vi "AI Regs Group UI.vi"(8 "error in (no error)":errorcluster, 11 "Node Ptr":T2 format="%.0x") -> (0 "error out":errorcluster)   [LabVIEW 2021, in "Modbus Master System Explorer.lvlib"]
uses:
  Modbus Master System Explorer.lvlib
  <vilib>/NI VeriStand/Custom Device API/Custom Device Item Ref.ctl
  SubVIs/Conflict Table.ctl
  SubVIs/Modbus Type.ctl
  <vilib>/NI VeriStand/Custom Device API/Custom Device API.lvlib
  <vilib>/NI VeriStand/Custom Device Tools/Custom Device Utility Library/Custom Device Utility Library.lvlib
  Shared/Modbus Master Shared.lvlib
panel:
  in  "Delete Multiple":bool
  in  "Add One":bool
  in  "Bulk Add":bool
  out "Conflicting Input Register Mappings":T1
  in  "Header":cluster{"Section Name":string}={"Section Name"="Input Register Group Settings"}
  in  "Description":string
  in  "Name":string
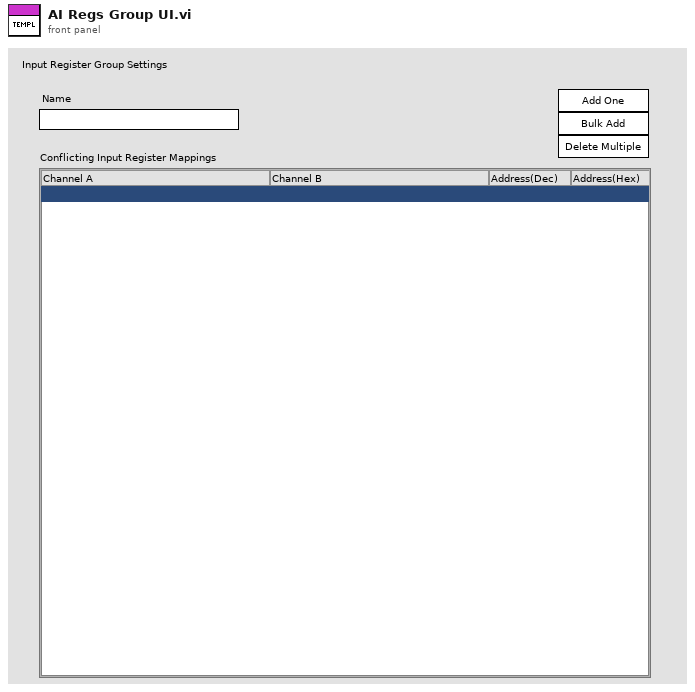
[diagram p1: front panel]
types:
  T1 = typedef "Modbus Master System Explorer.lvlib/Conflict Table.ctl" = i32
  T2 = typedef "Custom Device API.lvlib/Custom Device Item Ref.ctl" = u64
  T3 = typedef "Modbus Master Shared.lvlib/Modbus Type.ctl" = enum16{"Coil", "Discrete Input", "Holding Register", "Input Register"}
  T4 = typedef "Custom Device API.lvlib/Custom Device Item Info.ctl" = cluster{"Name":string, "Is Channel":bool, "GUID":string, "Is Waveform":bool}
  T5 = cluster{"Name":string, "Name":string, "Mapping":u16}[]
  T6 = typedef "Custom Device API.lvlib/Custom Device Commands.ctl" = enum16{"Default", "Item renamed", "Shutdown", "Dynamic button pressed"}
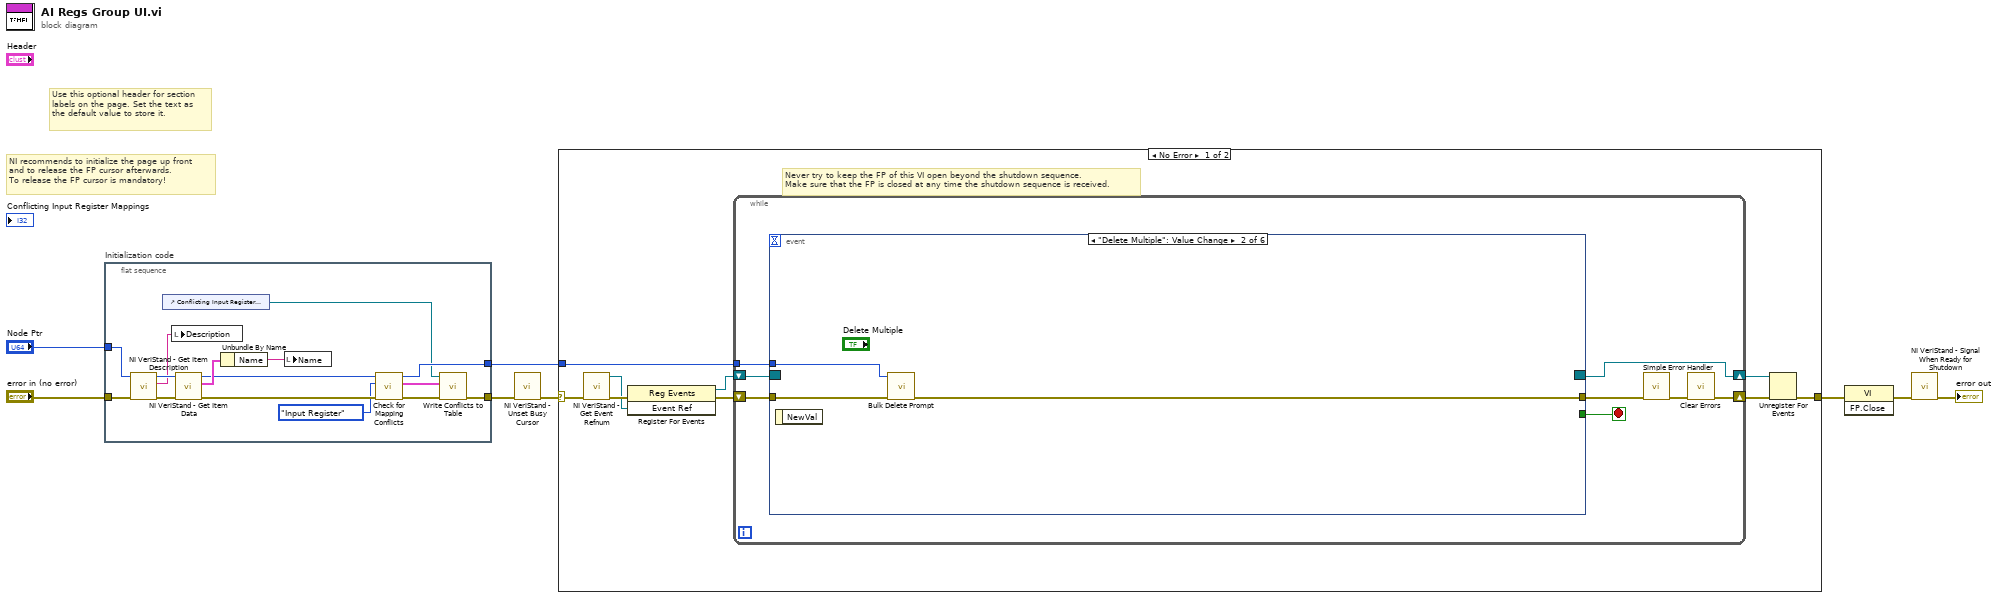
[diagram p0: block diagram]
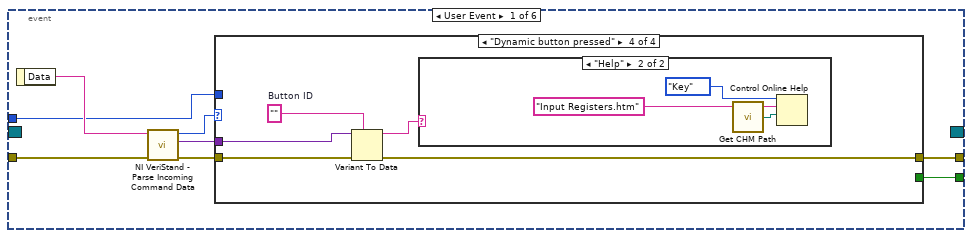
[diagram p2: hidden frame]
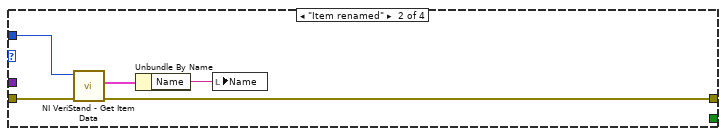
[diagram p4: hidden frame]
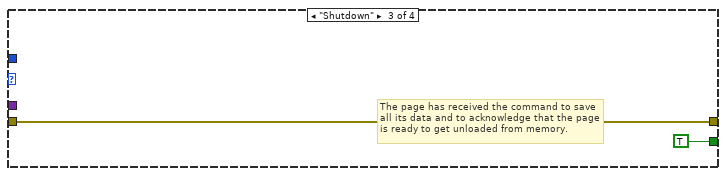
[diagram p5: hidden frame]
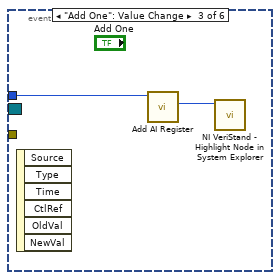
[diagram p7: hidden frame]
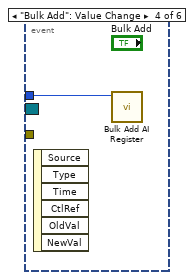
[diagram p8: hidden frame]
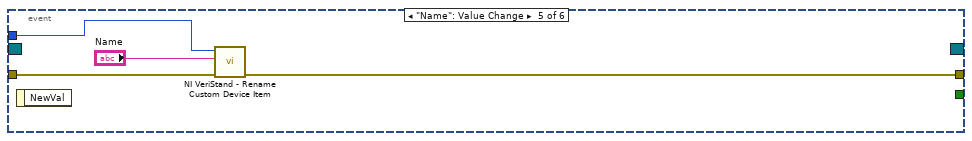
[diagram p9: hidden frame]
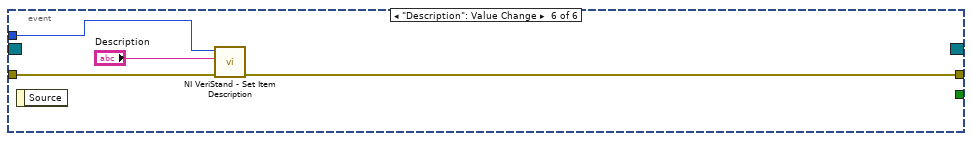
[diagram p10: hidden frame]
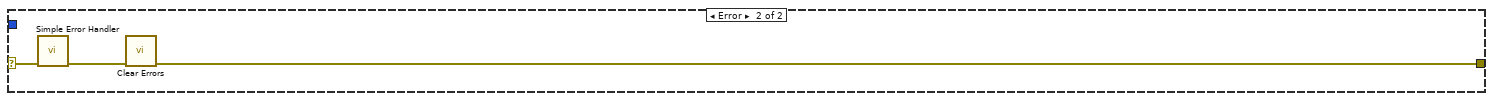
[diagram p11: hidden frame]
diagram:
  # "Use this optional header for section labels on the page. Set the text as the default value to store it."
  # "NI recommends to initialize the page up front\nand to release the FP cursor afterwards.\nTo release the FP cursor is mandatory!"
  n1 = flat-sequence "Initialization code" {
    tunnel: "error in (no error)" -> [w22]
    tunnel: "Node Ptr" -> [w21]
    tunnel: [w10] -> w4
    tunnel: [w15] -> w1
    frame #0 {
      n2 = call <vilib>:"NI VeriStand - Get Item Description.vi"("error in (no error)"=w22, "Item Ref in"=w21) -> ("error out"=w19:errorcluster, "Description"=w20:string, "Item Ref out"=w23:T2)  [unwired: 7 out]
      n3 = control-ref of="Conflicting Input Register Mappings"() -> (w13:refnum<vi>)
      n4 = local write "Description"(w20) -> ()
      n5 = call <vilib>:"NI VeriStand - Get Item Data.vi"("error in (no error)"=w19, "Item Ref in"=w23) -> ("error out"=w14:errorcluster, "Item Info"=w18:T4, "Item Ref out"=w16:T2)  [unwired: 7 out]
      n6 = Unbundle By Name(w18) -> ("Name"=w17:string)
      n7 = local write "Name"(w17) -> ()
      n8 = call "Check for Mapping Conflicts.vi"("error in (no error)"=w14, "Type"=Modbus_Type."Input Register", "Coiil Group Ref in in"=w16) -> ("error out"=w11:errorcluster, "Array"=w12:T5, "Coiil Group Ref out"=w15:T2)  [unwired: 5 in, 1 out]
      n9 = call "Write Conflicts to Table.vi"("error in (no error)"=w11, "Conflicts"=w12, "MC Listbox Ref"=w13) -> ("error out"=w10:errorcluster)  [unwired: 8 in]
    }
  }
  n10 = call <vilib>:"NI VeriStand - Unset Busy Cursor.vi"("error in (no error)"=w4) -> ("error out"=w3:errorcluster)  [unwired: 10 out]
  n11 = case shown="No Error" w3 {
    selector: w3 -> [w24 w81]
    tunnel: [w29 w79] -> w8
    tunnel: w1 -> [w25 _]
    frame No Error {
      # "Never try to keep the FP of this VI open beyond the shutdown sequence.\nMake sure that the FP is closed at any time the shutdown sequence is received."
      n12 = call <vilib>:"NI VeriStand - Get Event Refnum.vi"("error in (no error)"=w24) -> ("error out"=w32:errorcluster, "Event Ref"=w28:refnum<user-event>)  [unwired: 9 out]
      n13 = register-events(error in=w32, w28) -> (reference out=w26:refnum<event-registration>, error out=w27:errorcluster)  [unwired: 1 in]
      n14 = while {
        tunnel: w25 -> [w36]
        shift-right: [w33] -> w30
        shift-left: w27 -> [w39]
        shift-right: [w40] -> w31
        shift-left: w26 -> [w38]
        stop <- w37 stop-if-true
        n15 = event shown="[1] \"Delete Multiple\": Value Change" {
          selector: w38 -> [_ _ _ _ _ _]
          dyn-events: [_ _ _ _ _ _] -> w40
          timeout: _ -> [_ _ _ _ _ _]
          tunnel: w39 -> [w48 w66 _ _ w74 w77]
          tunnel: [w44 _ _ _ _ _] -> w37
          tunnel: [w43 w65 _ _ w73 w76] -> w35
          tunnel: w36 -> [w42 w67 w69 w70 w72 w78]
          event User Event {
            n16 = event-data() -> ("Data"=w47:string)  [unwired: 1 out]
            n17 = call <vilib>:"NI VeriStand - Parse Incoming Command Data.vi"("error in (no error)"=w48, "Incoming data"=w47) -> ("error out"=w46:errorcluster, "Outgoing data"=w41:variant, "Action"=w45:T6)  [unwired: 7 out]
            n18 = case shown="\"Dynamic button pressed\"" w45 {
              tunnel: w46 -> [w49 w54 w55 w61]
              tunnel: [_ _ TRUE _] -> w44
              tunnel: [w49 w51 w55 w58] -> w43
              tunnel: w42 -> [_ w53 _ _]
              tunnel: w41 -> [_ _ _ w60]
              frame "Default", Default {
              }
              frame "Item renamed" {
                n19 = call <vilib>:"NI VeriStand - Get Item Data.vi"("error in (no error)"=w54, "Item Ref in"=w53) -> ("error out"=w51:errorcluster, "Item Info"=w52:T4)  [unwired: 8 out]
                n20 = Unbundle By Name(w52) -> ("Name"=w50:string)
                n21 = local write "Name"(w50) -> ()
              }
              frame "Shutdown" {
                # "The page has received the command to save all its data and to acknowledge that the page is ready to get unloaded from memory."
              }
              frame "Dynamic button pressed" {
                w59 = ""  # Button ID
                n22 = Variant To Data(error in=w61, type=w59, Variant=w60) -> (data=w57:string, error out=w58:errorcluster)
                n23 = case shown="\"Help\"" w57 {
                  frame Default {
                  }
                  frame "Help" {
                    n24 = call "Get CHM Path.vi"() -> ("appended path"=w64:path)
                    n25 = Control Online Help(2:w64, 3:"Input Registers.htm" ("String to search for"), 4:enum16{"Contents", "Key", "Close"}."Key" ("Operation")) -> ()  [unwired: 1 in, 1 out]
                  }
                }
              }
            }
          }
          event "Delete Multiple": Value Change {
            n26 = event-data() -> ()  [unwired: 2 out]
            n27 = call "Bulk Delete Prompt.vi"("error in (no error)"=w66, "Item Ref in"=w67) -> ("error out"=w65:errorcluster)  [unwired: 9 in]
          }
          event "Add One": Value Change {
            n28 = event-data() -> ()  [unwired: 7 out]
            n29 = call "Add AI Register.vi"("Node Ref In"=w69) -> ("Channel Ref out"=w68:T2)  [unwired: 8 in, 2 out]
            n30 = call <vilib>:"NI VeriStand - Highlight Node in System Explorer.vi"("Item Ref in"=w68) -> ()  [unwired: 9 in, 2 out]
          }
          event "Bulk Add": Value Change {
            n31 = event-data() -> ()  [unwired: 7 out]
            n32 = call "Bulk Add AI Register.vi"("Node Ptr"=w70) -> ()  [unwired: 11 in]
          }
          event "Name": Value Change {
            n33 = event-data() -> ()  [unwired: 2 out]
            n34 = call <vilib>:"NI VeriStand - Rename Custom Device Item.vi"("error in (no error)"=w74, "New Name"="Name", "Item Ref in"=w72) -> ("error out"=w73:errorcluster)  [unwired: 1 in, 7 out]
          }
          event "Description": Value Change {
            n35 = event-data() -> ()  [unwired: 2 out]
            n36 = call <vilib>:"NI VeriStand - Set Item Description.vi"("error in (no error)"=w77, "Description"="Description", "Item Ref in"=w78) -> ("error out"=w76:errorcluster)  [unwired: 8 out]
          }
        }
        n37 = call <vilib>:"Simple Error Handler.vi"("error in (no error)"=w35) -> ("error out"=w34:errorcluster)  [unwired: 1 in, 7 out]
        n38 = call <vilib>:"Clear Errors.vi"("error in (no error)"=w34) -> ("error out"=w33:errorcluster)  [unwired: 1 in, 5 out]
      }
      n39 = Unregister For Events(event registration refnum=w31, error in=w30) -> (error out=w29:errorcluster)
    }
    frame Error {
      n40 = call <vilib>:"Simple Error Handler.vi"("error in (no error)"=w81) -> ("error out"=w80:errorcluster)  [unwired: 1 in, 7 out]
      n41 = call <vilib>:"Clear Errors.vi"("error in (no error)"=w80) -> ("error out"=w79:errorcluster)  [unwired: 1 in, 5 out]
    }
  }
  n42 = invoke class="VI" method="FP.Close"(error in=w8) -> (error out=w7:errorcluster)  [unwired: 2 in, 2 out]
  n43 = call <vilib>:"NI VeriStand - Signal When Ready for Shutdown.vi"("error in (no error)"=w7) -> ("error out"=→"error out":errorcluster)  [unwired: 10 out]
